vi "Display Animation.vi"(8 "error in (no error)":errorcluster, 10 "Animations":T1, 11 "Grove 2 RGB LED Matrix In":refnum<class "Grove 2 RGB LED Matrix.lvclass">) -> (0 "error out":errorcluster, 3 "Grove 2 RGB LED Matrix Out":refnum<class "Grove 2 RGB LED Matrix.lvclass">)   [LabVIEW 2020, in "CTI-Peripheral.lvlib" / "Grove 2 RGB LED Matrix.lvclass"]
uses:
  Grove 2 RGB LED Matrix.lvclass
  Data Types/Animations.ctl
  Grove 2 RGB LED Matrix.lvclass/Grove 2 RGB LED Matrix.ctl
  Data Types/MatrixI2CCommand.ctl
  CTI/I2C Connection/I2C Connection.lvclass/I2C Connection.ctl
  69a84970-3a55-48ac-9f7b-5110a78ebfc5.vi
  6387f02e-22fa-43de-95e8-1189edb91cdc.vi
  9b6cf815-83a5-41e0-be5c-301d7318f5b0.vi
  8f683837-54aa-459e-b131-6e7df6a372b6.vi
  CTI/Session/I2C Write Data.vi
  CTI/I2C Connection/I2C Connection.lvclass
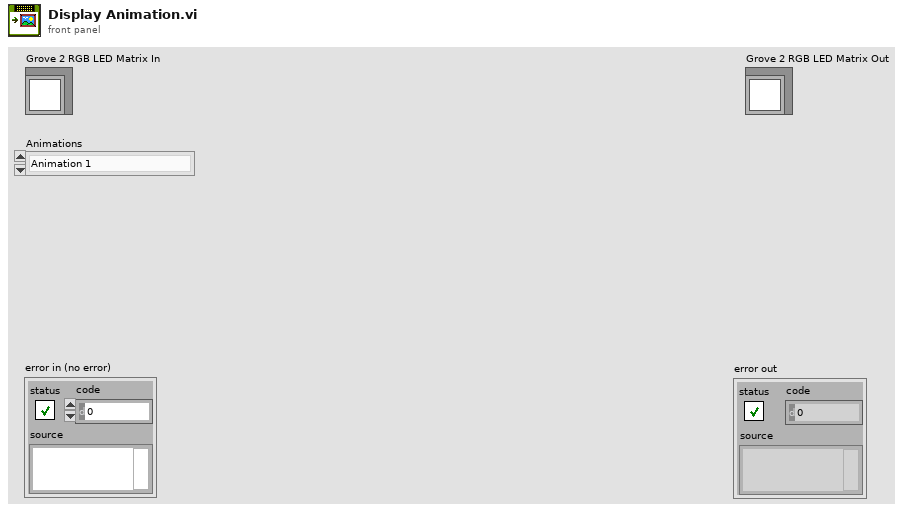
[diagram p1: front panel]
types:
  T1 = typedef "CTI-Peripheral.lvlib/Grove 2 RGB LED Matrix.lvclass/Animations.ctl" = enum16{"Animation 1", "Animation 2", "Rainbow Cycle", "Fire", "Walking", "Broken Heart"}
  T2 = typedef "CTI-Peripheral.lvlib/Grove 2 RGB LED Matrix.lvclass/MatrixI2CCommand.ctl" = u8
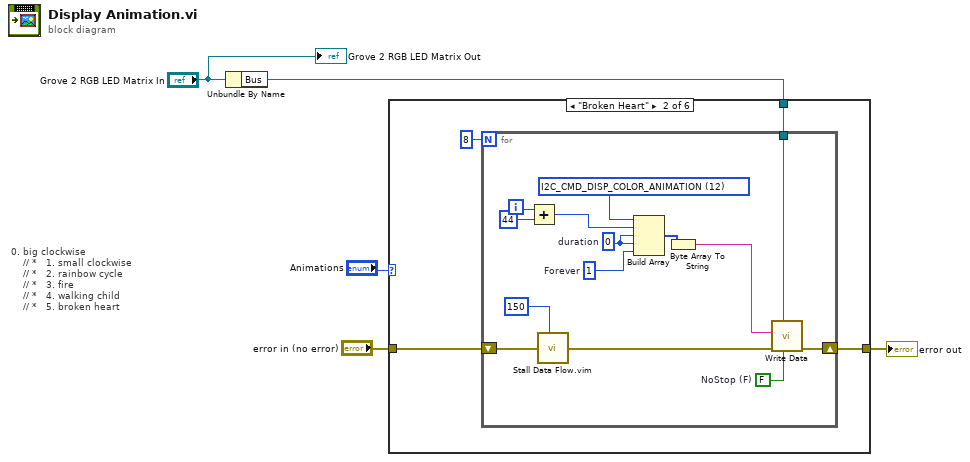
[diagram p0: block diagram]
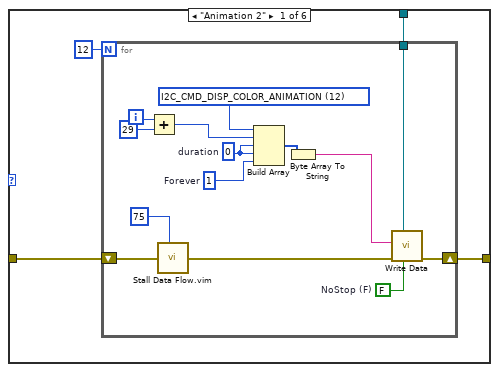
[diagram p2: hidden frame]
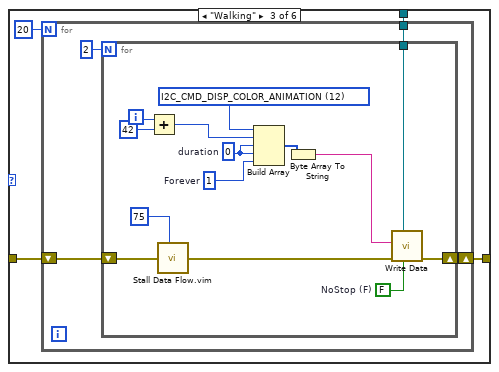
[diagram p3: hidden frame]
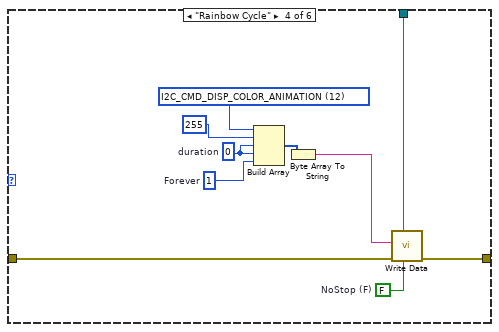
[diagram p4: hidden frame]
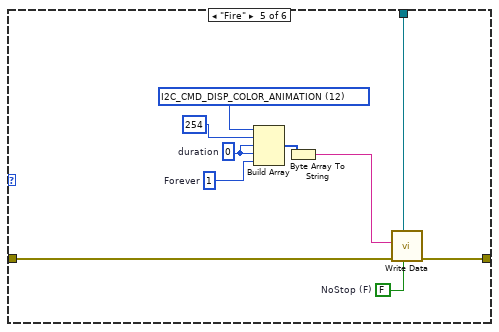
[diagram p5: hidden frame]
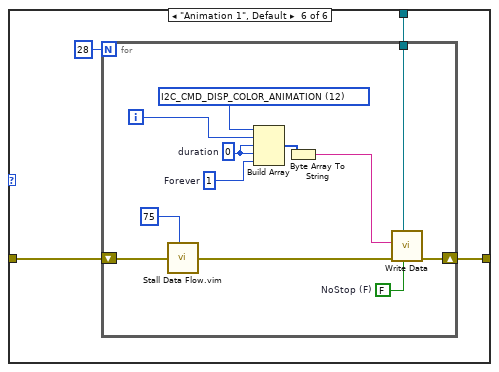
[diagram p6: hidden frame]
diagram:
  # "0. big clockwise\n    // *\t\t\t1. small clockwise\n    // *\t\t\t2. rainbow cycle\n    // *\t\t\t3. fire\n    // *\t\t\t4. walking child\n    // *\t\t\t5. broken heart"
  n1 = Unbundle By Name("Grove 2 RGB LED Matrix In") -> ("Bus"=w4:refnum<class "I2C Connection.lvclass">)
  n2 = case shown="\"Broken Heart\"" "Animations" {
    tunnel: w4 -> [w9 w27 w45 w73 w83 w87]
    tunnel: [w8 w26 w44 w72 w82 w86] -> w3
    tunnel: "error in (no error)" -> [w7 w25 w43 w71 w81 w85]
    frame "Animation 2" {
      n3 = for {
        N: 12 -> [_]
        tunnel: w9 -> [w17]
        shift-right: [w16] -> w8
        shift-left: w7 -> [w15]
        i -> [w14]
        w19 = u8 0  # duration
        w21 = FALSE  # NoStop (F)
        w18 = u8 1  # Forever
        w22 = T2 12 items=["I2C_CMD_GET_DEV_ID"=0, "I2C_CMD_DISP_BAR"=1, "I2C_CMD_DISP_EMOJI"=2, "I2C_CMD_DISP_NUM"=3, "I2C_CMD_DISP_STR"=4, "I2C_CMD_DISP_CUSTOM"=5, "I2C_CMD_DISP_OFF"=6, "I2C_CMD_DISP_ASCII"=7, "I2C_CMD_DISP_FLASH"=8, "I2C_CMD_DISP_COLOR_BAR"=9, "I2C_CMD_DISP_COLOR_WAVE"=10, "I2C_CMD_DISP_COLOR_CLOCKWISE"=11, "I2C_CMD_DISP_COLOR_ANIMATION"=12, "I2C_CMD_DISP_COLOR_BLOCK "=13, "I2C_CMD_STORE_FLASH"=160, "I2C_CMD_DELETE_FLASH"=161, "I2C_CMD_LED_ON"=176, "I2C_CMD_LED_OFF"=177, "I2C_CMD_AUTO_SLEEP_ON"=178, "I2C_CMD_AUTO_SLEEP_OFF"=179, "I2C_CMD_DISP_ROTATE"=180, "I2C_CMD_DISP_OFFSET"=181, "I2C_CMD_SET_ADDR"=192, "I2C_CMD_RST_ADDR"=193, "I2C_CMD_TEST_GET_VER"=226, "I2C_CMD_GET_DEVICE_UID"=241] ("I2C Command")
        n4 = Add(x=w14, y=29) -> (x+y=w12:i32)
        n5 = call "Stall Data Flow.vim"("value in"=w15, "milliseconds to wait"=u32 75) -> ("value out"=w11:errorcluster)  [unwired: 1 out]
        n6 = Build Array(w22, w12, w19, w19, w18) -> (w23:i32[])
        n7 = Byte Array To String(unsigned byte array=w23) -> (string=w20:string)
        n8 = call "Write Data.vi"("NoStop (F)"=w21, "I2C Connection"=w17, "error in (no error)"=w11, "Data"=w20) -> ("error out"=w16:errorcluster)  [unwired: 7 in]
      }
    }
    frame "Broken Heart" {
      n9 = for {
        N: 8 -> [_]
        tunnel: w27 -> [w35]
        shift-right: [w34] -> w26
        shift-left: w25 -> [w33]
        i -> [w32]
        w37 = u8 0  # duration
        w39 = FALSE  # NoStop (F)
        w36 = u8 1  # Forever
        w40 = T2 12 items=["I2C_CMD_GET_DEV_ID"=0, "I2C_CMD_DISP_BAR"=1, "I2C_CMD_DISP_EMOJI"=2, "I2C_CMD_DISP_NUM"=3, "I2C_CMD_DISP_STR"=4, "I2C_CMD_DISP_CUSTOM"=5, "I2C_CMD_DISP_OFF"=6, "I2C_CMD_DISP_ASCII"=7, "I2C_CMD_DISP_FLASH"=8, "I2C_CMD_DISP_COLOR_BAR"=9, "I2C_CMD_DISP_COLOR_WAVE"=10, "I2C_CMD_DISP_COLOR_CLOCKWISE"=11, "I2C_CMD_DISP_COLOR_ANIMATION"=12, "I2C_CMD_DISP_COLOR_BLOCK "=13, "I2C_CMD_STORE_FLASH"=160, "I2C_CMD_DELETE_FLASH"=161, "I2C_CMD_LED_ON"=176, "I2C_CMD_LED_OFF"=177, "I2C_CMD_AUTO_SLEEP_ON"=178, "I2C_CMD_AUTO_SLEEP_OFF"=179, "I2C_CMD_DISP_ROTATE"=180, "I2C_CMD_DISP_OFFSET"=181, "I2C_CMD_SET_ADDR"=192, "I2C_CMD_RST_ADDR"=193, "I2C_CMD_TEST_GET_VER"=226, "I2C_CMD_GET_DEVICE_UID"=241] ("I2C Command")
        n10 = Add(x=w32, y=44) -> (x+y=w30:i32)
        n11 = call "Stall Data Flow.vim"("value in"=w33, "milliseconds to wait"=u32 150) -> ("value out"=w29:errorcluster)  [unwired: 1 out]
        n12 = Build Array(w40, w30, w37, w37, w36) -> (w41:i32[])
        n13 = Byte Array To String(unsigned byte array=w41) -> (string=w38:string)
        n14 = call "Write Data.vi"("NoStop (F)"=w39, "I2C Connection"=w35, "error in (no error)"=w29, "Data"=w38) -> ("error out"=w34:errorcluster)  [unwired: 7 in]
      }
    }
    frame "Walking" {
      n15 = for {
        N: 20 -> [_]
        tunnel: w45 -> [w49]
        shift-right: [w48] -> w44
        shift-left: w43 -> [w47]
        n16 = for {
          N: 2 -> [_]
          tunnel: w49 -> [w57]
          shift-right: [w56] -> w48
          shift-left: w47 -> [w55]
          i -> [w54]
          w59 = u8 0  # duration
          w61 = FALSE  # NoStop (F)
          w58 = u8 1  # Forever
          w62 = T2 12 items=["I2C_CMD_GET_DEV_ID"=0, "I2C_CMD_DISP_BAR"=1, "I2C_CMD_DISP_EMOJI"=2, "I2C_CMD_DISP_NUM"=3, "I2C_CMD_DISP_STR"=4, "I2C_CMD_DISP_CUSTOM"=5, "I2C_CMD_DISP_OFF"=6, "I2C_CMD_DISP_ASCII"=7, "I2C_CMD_DISP_FLASH"=8, "I2C_CMD_DISP_COLOR_BAR"=9, "I2C_CMD_DISP_COLOR_WAVE"=10, "I2C_CMD_DISP_COLOR_CLOCKWISE"=11, "I2C_CMD_DISP_COLOR_ANIMATION"=12, "I2C_CMD_DISP_COLOR_BLOCK "=13, "I2C_CMD_STORE_FLASH"=160, "I2C_CMD_DELETE_FLASH"=161, "I2C_CMD_LED_ON"=176, "I2C_CMD_LED_OFF"=177, "I2C_CMD_AUTO_SLEEP_ON"=178, "I2C_CMD_AUTO_SLEEP_OFF"=179, "I2C_CMD_DISP_ROTATE"=180, "I2C_CMD_DISP_OFFSET"=181, "I2C_CMD_SET_ADDR"=192, "I2C_CMD_RST_ADDR"=193, "I2C_CMD_TEST_GET_VER"=226, "I2C_CMD_GET_DEVICE_UID"=241] ("I2C Command")
          n17 = Add(x=w54, y=42) -> (x+y=w52:i32)
          n18 = call "Stall Data Flow.vim"("value in"=w55, "milliseconds to wait"=u32 75) -> ("value out"=w51:errorcluster)  [unwired: 1 out]
          n19 = Build Array(w62, w52, w59, w59, w58) -> (w63:i32[])
          n20 = Byte Array To String(unsigned byte array=w63) -> (string=w60:string)
          n21 = call "Write Data.vi"("NoStop (F)"=w61, "I2C Connection"=w57, "error in (no error)"=w51, "Data"=w60) -> ("error out"=w56:errorcluster)  [unwired: 7 in]
        }
      }
    }
    frame "Rainbow Cycle" {
      w66 = u8 0  # duration
      w68 = FALSE  # NoStop (F)
      w65 = u8 1  # Forever
      w69 = T2 12 items=["I2C_CMD_GET_DEV_ID"=0, "I2C_CMD_DISP_BAR"=1, "I2C_CMD_DISP_EMOJI"=2, "I2C_CMD_DISP_NUM"=3, "I2C_CMD_DISP_STR"=4, "I2C_CMD_DISP_CUSTOM"=5, "I2C_CMD_DISP_OFF"=6, "I2C_CMD_DISP_ASCII"=7, "I2C_CMD_DISP_FLASH"=8, "I2C_CMD_DISP_COLOR_BAR"=9, "I2C_CMD_DISP_COLOR_WAVE"=10, "I2C_CMD_DISP_COLOR_CLOCKWISE"=11, "I2C_CMD_DISP_COLOR_ANIMATION"=12, "I2C_CMD_DISP_COLOR_BLOCK "=13, "I2C_CMD_STORE_FLASH"=160, "I2C_CMD_DELETE_FLASH"=161, "I2C_CMD_LED_ON"=176, "I2C_CMD_LED_OFF"=177, "I2C_CMD_AUTO_SLEEP_ON"=178, "I2C_CMD_AUTO_SLEEP_OFF"=179, "I2C_CMD_DISP_ROTATE"=180, "I2C_CMD_DISP_OFFSET"=181, "I2C_CMD_SET_ADDR"=192, "I2C_CMD_RST_ADDR"=193, "I2C_CMD_TEST_GET_VER"=226, "I2C_CMD_GET_DEVICE_UID"=241] ("I2C Command")
      n22 = Build Array(w69, 255 ("y"), w66, w66, w65) -> (w70:i32[])
      n23 = Byte Array To String(unsigned byte array=w70) -> (string=w67:string)
      n24 = call "Write Data.vi"("NoStop (F)"=w68, "I2C Connection"=w73, "error in (no error)"=w71, "Data"=w67) -> ("error out"=w72:errorcluster)  [unwired: 7 in]
    }
    frame "Fire" {
      w76 = u8 0  # duration
      w78 = FALSE  # NoStop (F)
      w75 = u8 1  # Forever
      w79 = T2 12 items=["I2C_CMD_GET_DEV_ID"=0, "I2C_CMD_DISP_BAR"=1, "I2C_CMD_DISP_EMOJI"=2, "I2C_CMD_DISP_NUM"=3, "I2C_CMD_DISP_STR"=4, "I2C_CMD_DISP_CUSTOM"=5, "I2C_CMD_DISP_OFF"=6, "I2C_CMD_DISP_ASCII"=7, "I2C_CMD_DISP_FLASH"=8, "I2C_CMD_DISP_COLOR_BAR"=9, "I2C_CMD_DISP_COLOR_WAVE"=10, "I2C_CMD_DISP_COLOR_CLOCKWISE"=11, "I2C_CMD_DISP_COLOR_ANIMATION"=12, "I2C_CMD_DISP_COLOR_BLOCK "=13, "I2C_CMD_STORE_FLASH"=160, "I2C_CMD_DELETE_FLASH"=161, "I2C_CMD_LED_ON"=176, "I2C_CMD_LED_OFF"=177, "I2C_CMD_AUTO_SLEEP_ON"=178, "I2C_CMD_AUTO_SLEEP_OFF"=179, "I2C_CMD_DISP_ROTATE"=180, "I2C_CMD_DISP_OFFSET"=181, "I2C_CMD_SET_ADDR"=192, "I2C_CMD_RST_ADDR"=193, "I2C_CMD_TEST_GET_VER"=226, "I2C_CMD_GET_DEVICE_UID"=241] ("I2C Command")
      n25 = Build Array(w79, 254 ("y"), w76, w76, w75) -> (w80:i32[])
      n26 = Byte Array To String(unsigned byte array=w80) -> (string=w77:string)
      n27 = call "Write Data.vi"("NoStop (F)"=w78, "I2C Connection"=w83, "error in (no error)"=w81, "Data"=w77) -> ("error out"=w82:errorcluster)  [unwired: 7 in]
    }
    frame "Animation 1", Default {
      n28 = for {
        N: 28 -> [_]
        tunnel: w87 -> [w93]
        shift-right: [w92] -> w86
        shift-left: w85 -> [w91]
        i -> [w90]
        w95 = u8 0  # duration
        w97 = FALSE  # NoStop (F)
        w94 = u8 1  # Forever
        w98 = T2 12 items=["I2C_CMD_GET_DEV_ID"=0, "I2C_CMD_DISP_BAR"=1, "I2C_CMD_DISP_EMOJI"=2, "I2C_CMD_DISP_NUM"=3, "I2C_CMD_DISP_STR"=4, "I2C_CMD_DISP_CUSTOM"=5, "I2C_CMD_DISP_OFF"=6, "I2C_CMD_DISP_ASCII"=7, "I2C_CMD_DISP_FLASH"=8, "I2C_CMD_DISP_COLOR_BAR"=9, "I2C_CMD_DISP_COLOR_WAVE"=10, "I2C_CMD_DISP_COLOR_CLOCKWISE"=11, "I2C_CMD_DISP_COLOR_ANIMATION"=12, "I2C_CMD_DISP_COLOR_BLOCK "=13, "I2C_CMD_STORE_FLASH"=160, "I2C_CMD_DELETE_FLASH"=161, "I2C_CMD_LED_ON"=176, "I2C_CMD_LED_OFF"=177, "I2C_CMD_AUTO_SLEEP_ON"=178, "I2C_CMD_AUTO_SLEEP_OFF"=179, "I2C_CMD_DISP_ROTATE"=180, "I2C_CMD_DISP_OFFSET"=181, "I2C_CMD_SET_ADDR"=192, "I2C_CMD_RST_ADDR"=193, "I2C_CMD_TEST_GET_VER"=226, "I2C_CMD_GET_DEVICE_UID"=241] ("I2C Command")
        n29 = call "Stall Data Flow.vim"("value in"=w91, "milliseconds to wait"=u32 75) -> ("value out"=w89:errorcluster)  [unwired: 1 out]
        n30 = Build Array(w98, w90, w95, w95, w94) -> (w99:i32[])
        n31 = Byte Array To String(unsigned byte array=w99) -> (string=w96:string)
        n32 = call "Write Data.vi"("NoStop (F)"=w97, "I2C Connection"=w93, "error in (no error)"=w89, "Data"=w96) -> ("error out"=w92:errorcluster)  [unwired: 7 in]
      }
    }
  }
  "error out" <- w3
  "Grove 2 RGB LED Matrix Out" <- "Grove 2 RGB LED Matrix In"
